vi "Stop Logging.vi"(8 "error in (no error)":errorcluster, 11 "Data Logger Interface in":refnum<class "Data Logger Actor Interface.lvclass">) -> (0 "error out":errorcluster, 3 "Data Logger Interface out":refnum<class "Data Logger Actor Interface.lvclass">)   [LabVIEW 2024, in "Data Logger Actor Interface.lvlib" / "Data Logger Actor Interface.lvclass"]
uses:
  Data Logger Actor Interface.lvclass
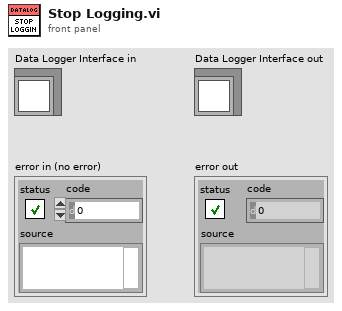
[diagram p1: front panel]
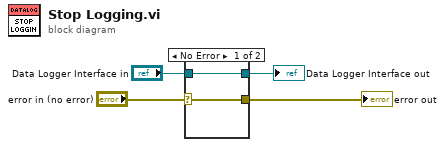
[diagram p0: block diagram]
diagram:
  n1 = case shown="No Error" "error in (no error)" {
    selector: "error in (no error)" -> [w5 w8]
    tunnel: [w5 w8] -> w3
    tunnel: [w6 w7] -> w1
    tunnel: "Data Logger Interface in" -> [w6 w7]
    frame No Error {
    }
    frame Error {
    }
  }
  "error out" <- w3
  "Data Logger Interface out" <- w1
